vi "Read Tag Name.vi"(8 "error in (no error)":errorcluster, 11 "Update Tag in":refnum<class "Update Tag Config.lvclass">) -> (0 "error out":errorcluster, 2 "Tag Name":string, 3 "Update Tag out":refnum<class "Update Tag Config.lvclass">)   [LabVIEW 2015]
uses:
  Update Tag Config.lvclass
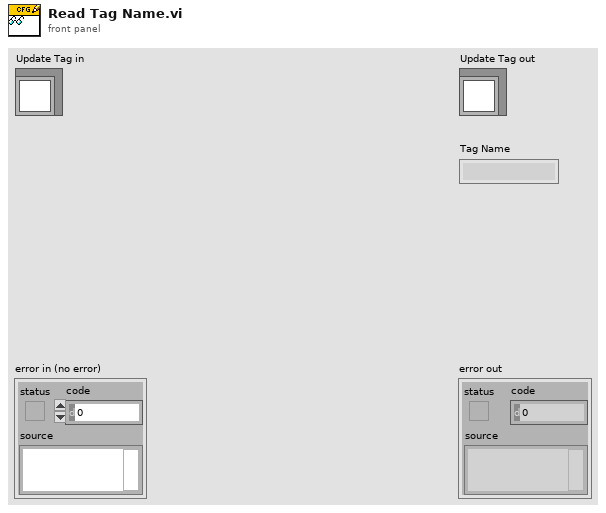
[diagram p1: front panel]
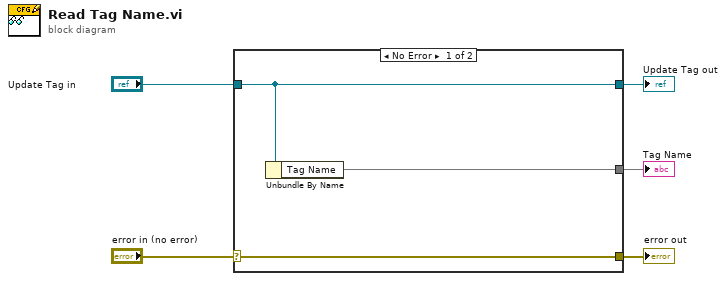
[diagram p0: block diagram]
diagram:
  n1 = case shown="No Error" "error in (no error)" {
    selector: "error in (no error)" -> [w8 w9]
    tunnel: [w8 w9] -> w4
    tunnel: [w7 w10] -> w2
    tunnel: "Update Tag in" -> [w7 w10]
    tunnel: [w6 _] -> w1
    frame No Error {
      n2 = Unbundle By Name(w7) -> ("Tag Name"=w6)
    }
    frame Error {
    }
  }
  "error out" <- w4
  "Update Tag out" <- w2
  "Tag Name" <- w1
